vi "Calculate RelativeX Samples.vi"(0 "fetch relative to":T1, 5 "pretrigger samples":u64, 7 "timestamps":dbl, 9 "fetch offset":i64) -> (4 "relativeX (samples)":dbl)   [LabVIEW 2021, in "Device Session.lvclass"]
uses:
  Device Session.lvclass
  <instrlib>/_niInstr/Multirecord Acquisition/Interface/v1/Host/Public/Fetch Relative To Enum.ctl
  <instrlib>/_niInstr/Multirecord Acquisition/Interface/v1/Host/niInstr Multirecord Acquisition v1 Host.lvclass
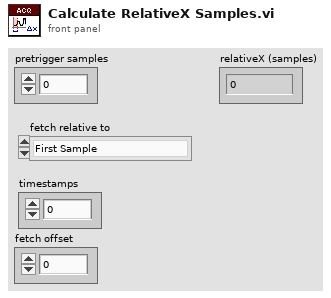
[diagram p1: front panel]
types:
  T1 = typedef "niInstr Multirecord Acquisition v1 Host.lvclass/Fetch Relative To Enum.ctl" = enum16{"First Sample", "Reference Trigger Sample", "First Pretrigger Sample", "Most Recent Sample", "Current Read Position"}
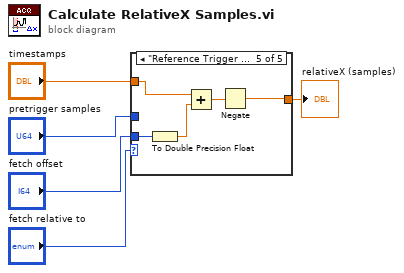
[diagram p0: block diagram]
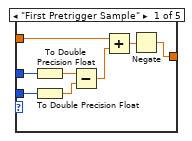
[diagram p2: hidden frame]
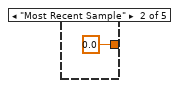
[diagram p3: hidden frame]
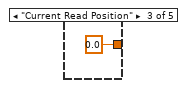
[diagram p4: hidden frame]
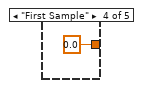
[diagram p5: hidden frame]
diagram:
  n1 = case shown="\"Reference Trigger Sample\"" "fetch relative to" {
    tunnel: "timestamps" -> [w9 _ _ _ w19]
    tunnel: [w6 0.0 0.0 0.0 w17] -> w1
    tunnel: "fetch offset" -> [w11 _ _ _ w21]
    tunnel: "pretrigger samples" -> [w12 _ _ _ _]
    frame "First Pretrigger Sample" {
      n2 = To Double Precision Float(number=w12) -> (double precision float=w13:dbl)
      n3 = To Double Precision Float(number=w11) -> (double precision float=w10:dbl)
      n4 = Subtract(x=w13, y=w10) -> (x-y=w8:dbl)
      n5 = Add(x=w9, y=w8) -> (x+y=w7:dbl)
      n6 = Negate(x=w7) -> (-x=w6:dbl)
    }
    frame "Most Recent Sample" {
    }
    frame "Current Read Position" {
    }
    frame "First Sample" {
    }
    frame "Reference Trigger Sample" {
      n7 = To Double Precision Float(number=w21) -> (double precision float=w20:dbl)
      n8 = Add(x=w19, y=w20) -> (x+y=w18:dbl)
      n9 = Negate(x=w18) -> (-x=w17:dbl)
    }
  }
  "relativeX (samples)" <- w1
